vi "Set Multiple Object Items.vi"(5 "Item Names":string[](array[string]), 6 "$Path or Item Name":string caption="Object $Path or Item Name", 7 "error in (no error)":errorcluster, 8 "JSON Items":string[](array[string]), 9 "Object Offset":i32, 10 "JSON":string="{}") -> (0 "error out":errorcluster, 3 "<JSON>":string)   [LabVIEW 2019, in "JSONtext.lvlib"]
doc: "Insert (or replace) multiple items into a JSON Object specified by the Object $Path. \n\nIf the path specified does not exist, but its immediate parent does, then a new object is created."
uses:
  JSONtext.lvlib
  Parsing/Found Items.ctl
  Parsing/Parsing State.ctl
  support/quote and escape json string 2.vi
  Parsing/Advance past whitespace.vi
  Parsing/Advance past whitespace and comma.vi
  Parsing/Advance past next JSON Value (inlined COPY).vi
  Parsing/Advance past Item Name.vi
  JDP Science Common Utilities/Trim Whitespace__JDP.vi
  Parsing/Advance past Line Ending.vi
  Parsing/Advance past String.vi
  Parsing/Advance past Number.vi
  Parsing/Advance past Array.vi
  Parsing/Advance past Object.vi
  Parsing/Parsing Error.vi
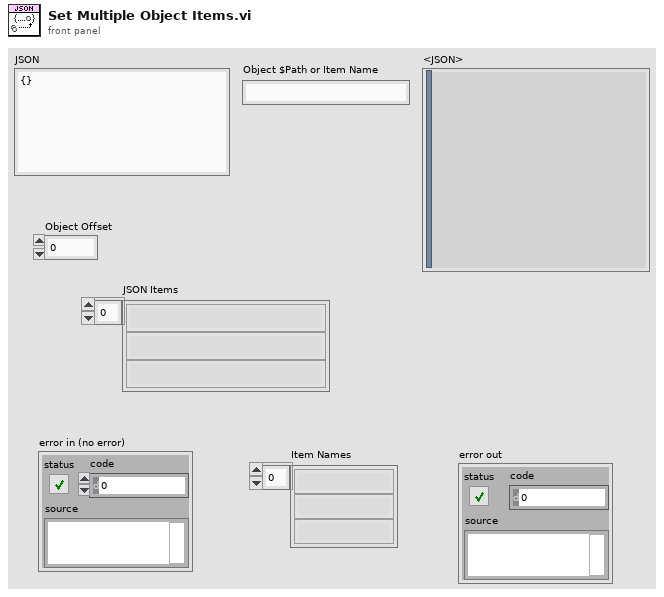
[diagram p1: front panel]
types:
  T1 = typedef "JSONtext.lvlib/Found Items.ctl" = cluster{"Item offset":i32, "Offset past Item":i32, "Name offset":i32, "Offset past Name":i32, "Found":bool, "Item Type":T2, "Item Index":i32, "Start Offset":i32, "Comma Needed For Insert":bool}
  T2 = typedef "JSONtext.lvlib/Parsing State.ctl" = enum16{"Parser Error", "Object", "Array", "String", "Number/Other", "Leading Whitespace", "Object end", "Array end", "Value end"}
  T3 = cluster{"Item":T1, "<JSON>Name":string, "<JSON>":string}
  T4 = cluster{"Item":T1, "<JSON>Name":string, "<JSON>":string}[]
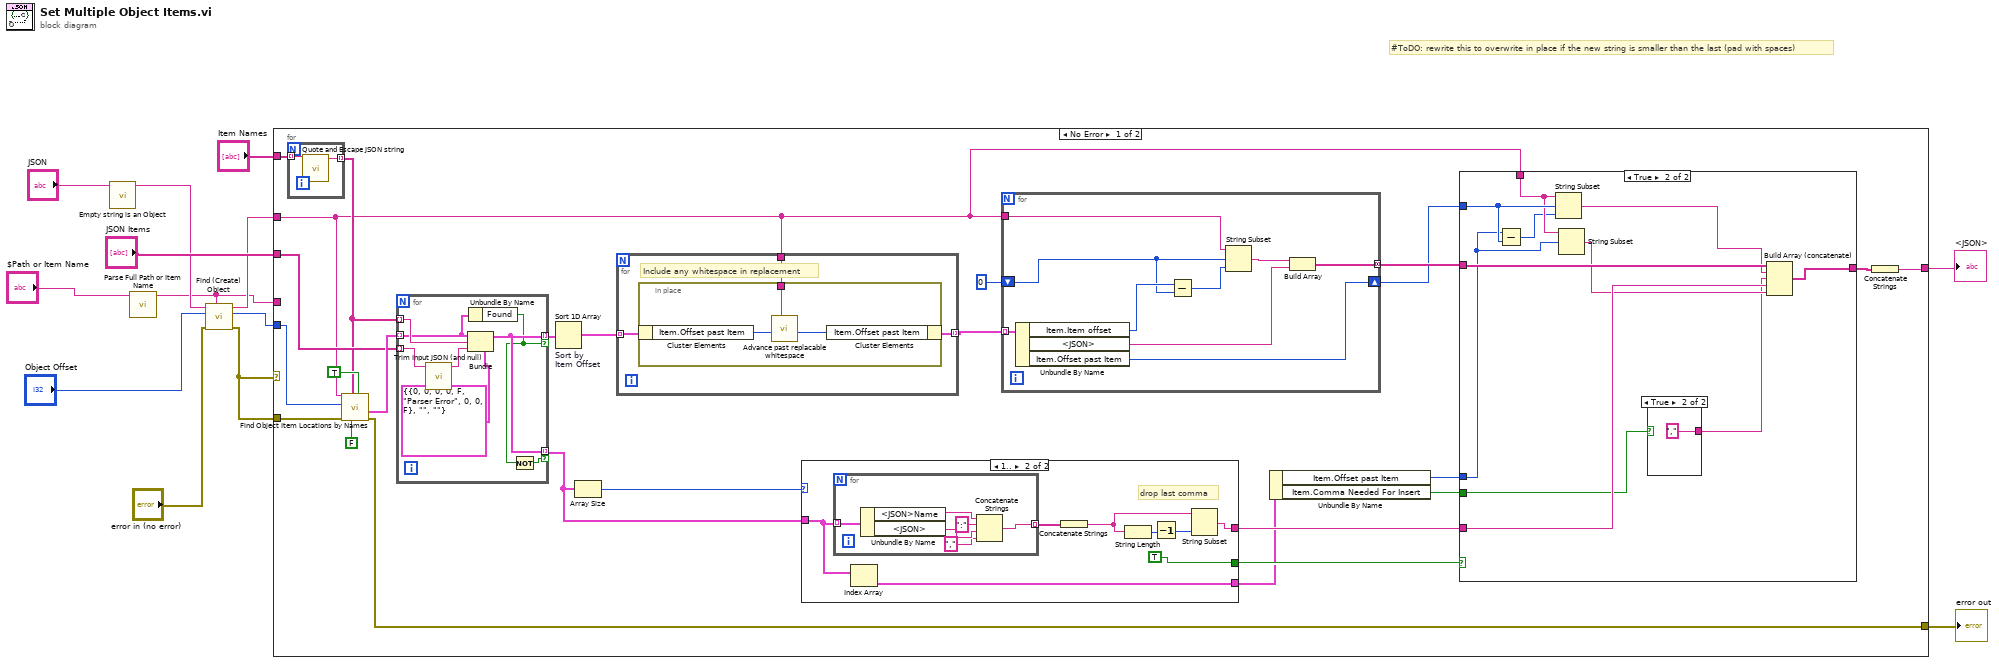
[diagram p0: block diagram]
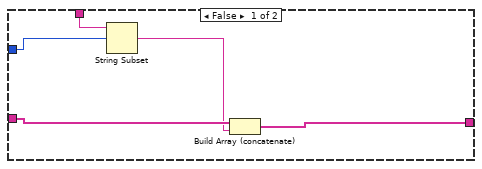
[diagram p2: hidden frame]
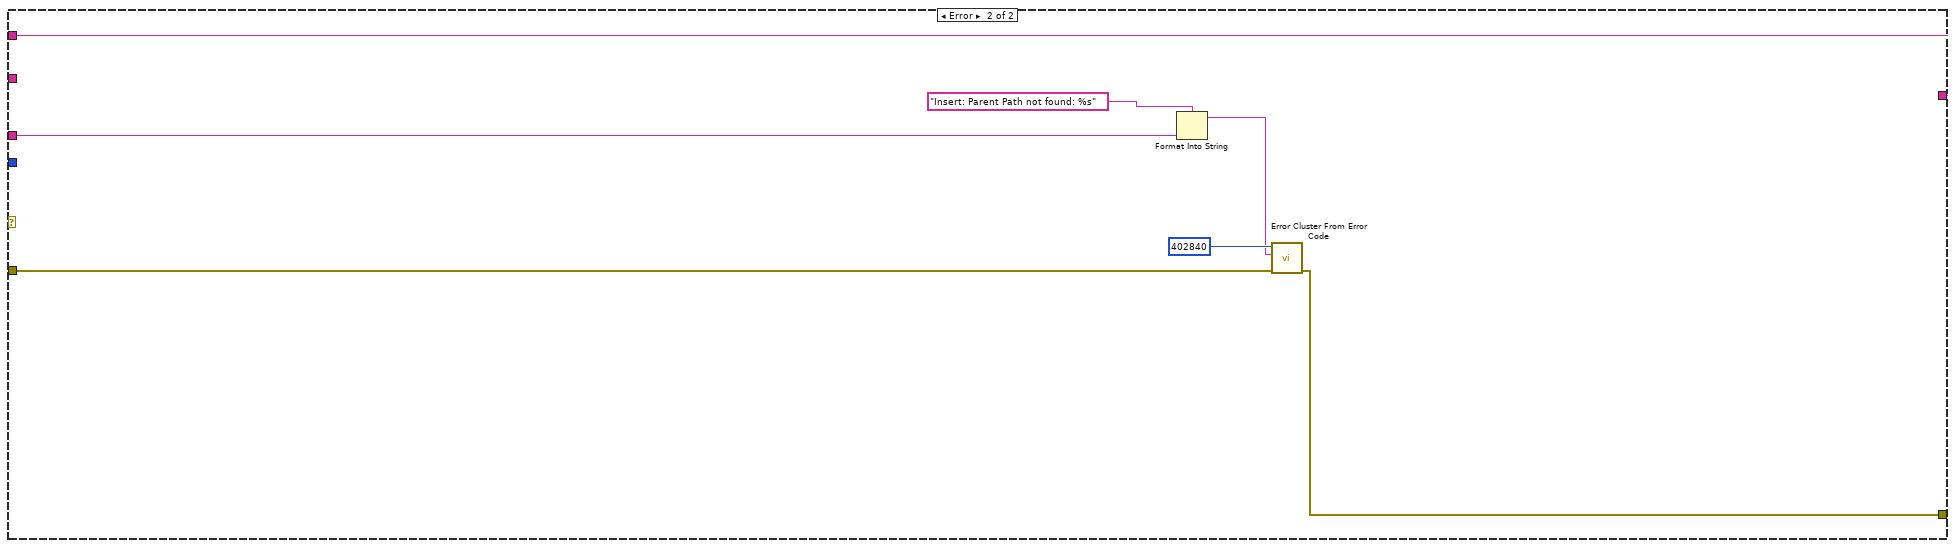
[diagram p5: hidden frame]
diagram:
  # "#ToDO: rewrite this to overwrite in place if the new string is smaller than the last (pad with spaces)"
  n1 = call "Empty string is an Object.vi"("JSON Input"="JSON") -> ("<JSON>Object"=w3:string)  [unwired: 10 in]
  n2 = call "Parse Full Path or Item Name.vi"("Full Path (with $) or Name"="$Path or Item Name") -> ("Relative Path or JSON-format name"=w2:string)  [unwired: 10 in]
  n3 = call "Find (Create) Object.vi"("Object Path"=w2, "error in (no error)"="error in (no error)", "Starting Offset"="Object Offset", "JSON"=w3) -> ("error out"=w5:errorcluster, "Object offset"=w11:i32, "<JSON>"=w7:string)  [unwired: 5 in]
  n4 = case shown="No Error" w5 {
    tunnel: "JSON Items" -> [w29 _]
    tunnel: w5 -> [w38 w95]
    tunnel: [w37 w100] -> w13
    tunnel: w7 -> [w15 w101]
    tunnel: w11 -> [w36 _]
    tunnel: "Item Names" -> [w35 _]
    tunnel: [w21 w101] -> w8
    tunnel: w2 -> [_ w96]
    frame No Error {
      n5 = for {
        tunnel: w35 -> [w94] mode=indexing
        tunnel: [w93] -> w27 mode=indexing
        n6 = call "Quote and Escape JSON string.vi"("Plain Text"=w94) -> ("<JSON>"=w93:string)  [unwired: 10 in]
      }
      n7 = call "Find Object Item Locations by Names.vi"("Insertion point if not found"=TRUE, "Only return first found"=FALSE, "Item Names <JSON>"=w27, "error in (no error)"=w38, "Object Offset"=w36, "JSON"=w15) -> ("error out"=w37:errorcluster, "Items"=w31:T1[])  [unwired: 4 in]
      n8 = for {
        tunnel: [w90] -> w32 mode=indexing if=w88
        tunnel: w31 -> [w91] mode=indexing
        tunnel: w27 -> [w92] mode=indexing
        tunnel: w29 -> [w87] mode=indexing
        tunnel: [w90] -> w26 mode=indexing if=w89
        n9 = call "Trim Input JSON (and null).vi"("JSON Input"=w87) -> ("<JSON>"=w86:string)  [unwired: 10 in]
        n10 = Bundle(cluster=T3 {"Item"={"Item offset"=0, "Offset past Item"=0, "Name offset"=0, "Offset past Name"=0, "Found"=FALSE, "Item Type"=enum."Parser Error", "Item Index"=0, "Start Offset"=0, "Comma Needed For Insert"=FALSE}, "<JSON>Name"="", "<JSON>"=""}, "Item"=w91, "<JSON>Name"=w92, "<JSON>"=w86) -> (w90:T3)
        n11 = Unbundle By Name(w91) -> ("Found"=w88:bool)
        n12 = Not(x=w88) -> (.not. x?=w89:bool)
      }
      n13 = Sort 1D Array "Sort by \nItem Offset"(array=w32) -> (sorted array=w30:T4)
      n14 = Array Size(array=w26) -> (size(s)=w25:i32)
      n15 = for {
        tunnel: w30 -> [w72] mode=indexing
        tunnel: [w71] -> w28 mode=indexing
        tunnel: w15 -> [w70]
        # "Include any whitespace in replacement"
        n16 = in-place {
          in-place-border: w70 -> [w74]
          n17 = in-place-cluster #1(w72) -> ("Item.Offset past Item"=w75:i32)
          n18 = call "Advance past replacable whitespace.vi"("JSON"=w74, "Offset"=w75) -> ("Offset of first non-whitespace"=w73:i32)  [unwired: 9 in]
          n19 = in-place-cluster #1("Item.Offset past Item"=w73) -> (w71:T3)
        }
      }
      n20 = case shown="1.." w25 {
        tunnel: w26 -> [_ w63]
        tunnel: [_ w62] -> w18
        tunnel: [_ w58] -> w22
        tunnel: [_ TRUE] -> w24
        frame 0, Default {
        }
        frame 1.. {
          # "drop last comma"
          n21 = for {
            tunnel: w63 -> [w69] mode=indexing
            tunnel: [w67] -> w57 mode=indexing
            n22 = Unbundle By Name(w69) -> ("<JSON>Name"=w66:string, "<JSON>"=w65:string)
            n23 = Concatenate Strings(w66, ":" ("string"), w65, "," ("delimiter (Tab)")) -> (w67:string)
          }
          n24 = Index Array(array=w63) -> (element=w62:T3)  [unwired: 1 in]
          n25 = Concatenate Strings(w57) -> (w56:string)
          n26 = String Length(string=w56) -> (length=w60:i32)
          n27 = Decrement(x=w60) -> (x-1=w59:i32)
          n28 = String Subset(string=w56, length (rest)=w59) -> (substring=w58:string)  [unwired: 1 in]
        }
      }
      n29 = for {
        tunnel: w15 -> [w82]
        tunnel: w28 -> [w84] mode=indexing
        tunnel: [w80] -> w23 mode=concatenating
        shift-right: [w79] -> w19
        shift-left: 0 ("Offset\nAdjustment") -> [w77]
        n30 = Unbundle By Name(w84) -> ("Item.Item offset"=w78:i32, "<JSON>"=w81:string, "Item.Offset past Item"=w79:i32)
        n31 = Subtract(x=w78, y=w77) -> (x-y=w76:i32)
        n32 = String Subset(string=w82, offset (0)=w77, length (rest)=w76) -> (substring=w83:string)
        n33 = Build Array(w83, w81) -> (w80:string[])
      }
      n34 = Unbundle By Name(w18) -> ("Item.Offset past Item"=w17:i32, "Item.Comma Needed For Insert"=w14:bool)
      n35 = case shown="True" w24 {
        tunnel: w23 -> [w43 w54]
        tunnel: w22 -> [_ w52]
        tunnel: [w40 w53] -> w16
        tunnel: w15 -> [w42 w50]
        tunnel: w19 -> [w41 w51]
        tunnel: w17 -> [_ w47]
        tunnel: w14 -> [_ w44]
        frame False {
          n36 = String Subset(string=w42, offset (0)=w41) -> (substring=w39:string)  [unwired: 1 in]
          n37 = Build Array (concatenate)(w43, w39) -> (w40:string[])
        }
        frame True {
          n38 = Subtract(x=w47, y=w51) -> (x-y=w49:i32)
          n39 = String Subset(string=w50, offset (0)=w51, length (rest)=w49) -> (substring=w46:string)
          n40 = String Subset(string=w50, offset (0)=w47) -> (substring=w48:string)  [unwired: 1 in]
          n41 = case shown="True" w44 {
            tunnel: [_ "," ("element")] -> w45
            frame False {
            }
            frame True {
            }
          }
          n42 = Build Array (concatenate)(w54, w46, w45, w52, w48) -> (w53:string[])
        }
      }
      n43 = Concatenate Strings(w16) -> (w21:string)
    }
    frame Error {
      n44 = Format Into String(format string="Insert: Parent Path not found: %s" ("error message (\"\")"), w96) -> (resulting string=w98:string)  [unwired: 2 in, 1 out]
      n45 = call <vilib>:"Error Cluster From Error Code.vi"("error in (no error)"=w95, "error message (\"\")"=w98, "error code (0)"=402840) -> ("error out"=w100:errorcluster)  [unwired: 6 in]
    }
  }
  "<JSON>" <- w8
  "error out" <- w13
